vi "V4fit.vi"(3 "output control":T2, 4 "data":T1, 5 "X":dbl[](array[numeric]), 6 "a":dbl[](array[numeric])) -> (0 "error out":errorcluster, 1 "f'(X,a)":dbl[][](array[numeric]), 2 "f(X,a)":dbl[](array[numeric]))   [LabVIEW 2018]
doc: "This template is the starting point for creating a model function to be passed to the Nonlinear Curve Fit.vi."
uses:
  <vilib>/gmath/NumericalOptimization/LM_output select.ctl
  <vilib>/gmath/NumericalOptimization/objective function data.ctl
  <vilib>/gmath/NI_Gmath.lvlib
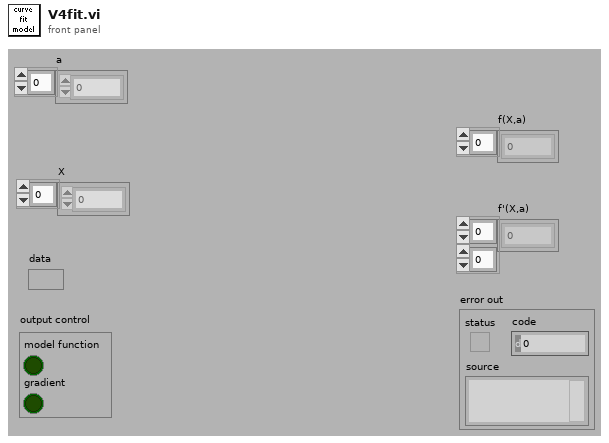
[diagram p1: front panel]
types:
  T1 = typedef "NI_Gmath.lvlib/objective function data.ctl" = variant
  T2 = typedef "NI_Gmath.lvlib/LM_output select.ctl" = cluster{"model function":bool, "gradient":bool}
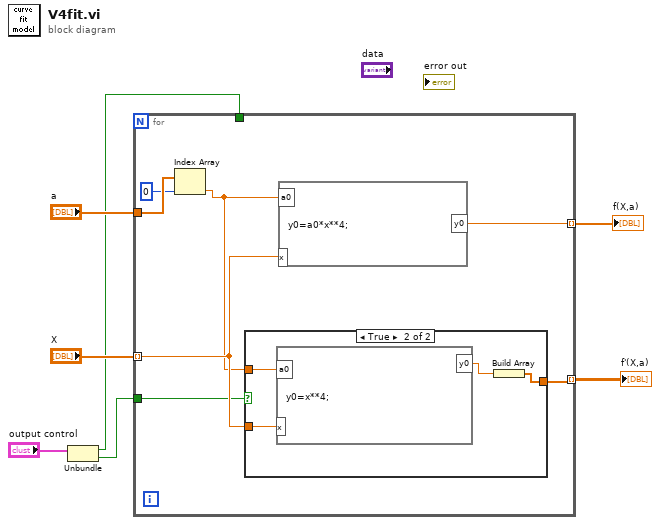
[diagram p0: block diagram]
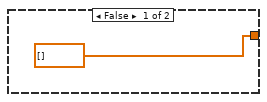
[diagram p2: hidden frame]
diagram:
  n1 = Unbundle("output control") -> ("model function"=w1:bool, "gradient"=w2:bool)
  n2 = for {
    tunnel: "a" -> [w12]
    tunnel: "X" -> [w14] mode=indexing
    tunnel: [w13] -> w5 mode=indexing
    tunnel: [w8] -> w4 mode=indexing
    tunnel: w2 -> [w9]
    tunnel: w1 -> [_]
    n3 = Index Array(array=w12, index=0) -> (element=w10:dbl)
    n4 = case shown="True" w9 {
      tunnel: w14 -> [_ w19]
      tunnel: w10 -> [_ w18]
      tunnel: [dbl[] [] w16] -> w8
      frame False {
      }
      frame True {
        n5 = formula code="y0=x**4;"("x"=w19, "a0"=w18) -> ("y0"=w17:dbl)
        n6 = Build Array(w17) -> (w16:dbl[])
      }
    }
    n7 = formula code="y0=a0*x**4;"("x"=w14, "a0"=w10) -> ("y0"=w13:dbl)
  }
  "f(X,a)" <- w5
  "f'(X,a)" <- w4
